vi "read write modules.vi"() -> ()   [LabVIEW 2017]
doc: "This vi simply calls all the modules with the normal connector pattern. It reads or writes the modules depending on the buttons inside each modules, or alternatively the global buttons for reading or writing ALL modules."
uses:
  globals/Modules global.vi
panel:
  out "Module number":i32
  out "appended path":path=path "modules and sub-vi's/Utility Module 01.vi"
  out "Module":u16(ring)=14 items=["Atom removal 1", "Atom removal 2", "B-field off", "CMOT", "Defaults", "Final B-field ramps", "Fluorescence pulse", "High field", "High field ARP", "Loading cart QT", "Loading sci QT", "Low field", "Low field ARP", "Mol OD image", "Mol picture", "Mol probe pulse", "Molasses", "MOT off", "MOT on", "OD image", "Optical pumping", "OT B-field off", "Picture", "Probe pulse", "QT off for OT", "Quadrupole trap off", "Quadrupole trap", "Quantization axis", "S-G separation", "STIRAP back for imaging", "STIRAP", "TTL high", "TTL low", "GPIB", "Utility Module 1", "Utility Module 2", "Utility Module 3", "Utility Module 4", "Utility Module 5", "Utility Module 6", "Utility Module 7", "Utility Module 8", "Utility Module 9"]
  in  "VI Type Specifier":refnum<vi>
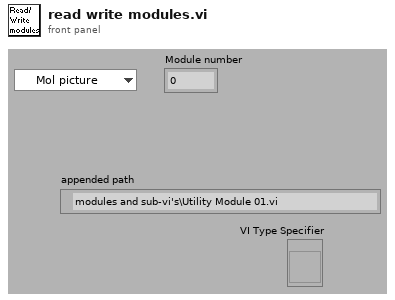
[diagram p1: front panel]
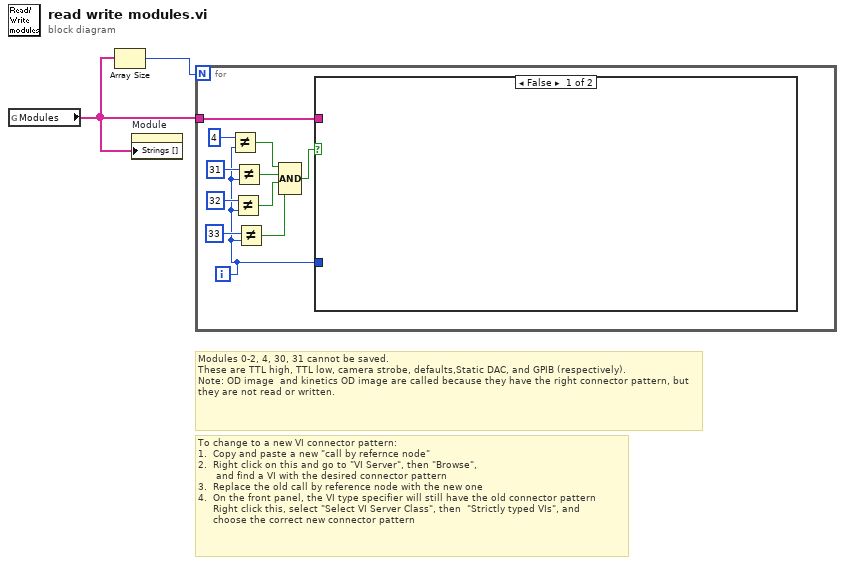
[diagram p0: block diagram]
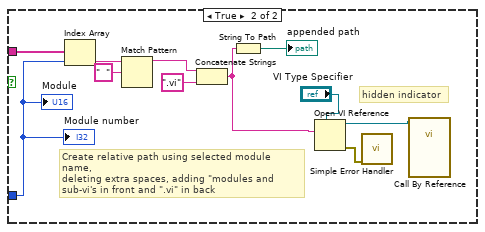
[diagram p2: hidden frame]
diagram:
  # "To change to a new VI connector pattern: \n1.  Copy and paste a new \"call by refernce node\"\n2.  Right click on this and go to \"VI Server\", then \"Browse\",\n      and find a VI with the desired connector pattern\n3.  Replace the old call by reference node with the new one\n4.  On the front panel, the VI type specifier will still have the old connector pattern\n     Right click this, select \"Select VI Server Class\", then  \"Strictly typed VIs\", and\n     choose the correct new connector pattern"
  # "Modules 0-2, 4, 30, 31 cannot be saved.\nThese are TTL high, TTL low, camera strobe, defaults,Static DAC, and GPIB (respectively).\nNote: OD image  and kinetics OD image are called because they have the right connector pattern, but\nthey are not read or written."
  n1 = global read "Modules global.vi" "Modules"() -> (w2:string[])
  n2 = Array Size(array=w2) -> (size(s)=w1:i32)
  n3 = property on="Module" class="Ring (strict)"("Strings []"=w2) -> ()  [unwired: 2 in, 2 out]
  n4 = for {
    N: w1 -> [_]
    tunnel: w2 -> [w13]
    i -> [w8]
    n5 = Not Equal?(x=u16 4 ("y"), y=w8) -> (x != y?=w7:bool)
    n6 = Not Equal?(x=u16 32 ("y"), y=w8) -> (x != y?=w5:bool)
    n7 = Not Equal?(x=u16 31 ("y"), y=w8) -> (x != y?=w6:bool)
    n8 = Not Equal?(x=u16 33 ("y"), y=w8) -> (x != y?=w4:bool)
    n9 = Compound Arithmetic op=AND(w7, w6, w5, w4) -> (w3:bool)
    n10 = case shown="False" w3 {
      tunnel: w13 -> [_ w20]
      tunnel: w8 -> [_ w19]
      frame False {
      }
      frame True {
        # "Create relative path using selected module name,\ndeleting extra spaces, adding \"modules and sub-vi's in front and \".vi\" in back"
        # "hidden indicator"
        n11 = Index Array(array=w20, index=w19) -> (element=w22:string)
        n12 = Match Pattern(string=w22, regular expression="  ") -> (before substring=w21:string)  [unwired: 1 in, 3 out]
        n13 = Concatenate Strings(w21, ".vi" ("Substring")) -> (w16:string)
        n14 = String To Path(string=w16) -> (path=→"appended path":path)
        n15 = Open VI Reference(type specifier VI Refnum (for type only)="VI Type Specifier", vi path=w16) -> (vi reference=w15:refnum<vi>, error out=w14:errorcluster)  [unwired: 4 in]
        n16 = call <vilib>:"Simple Error Handler.vi"("error in (no error)"=w14) -> ()  [unwired: 4 in, 5 out]
        n17 = call-by-ref "?"(reference=w15) -> ()  [unwired: 6 in, 5 out]
        "Module" <- w19
        "Module number" <- w19
      }
    }
  }
